vi "Write Recipe Data.vi"(8 "error in (no error)":errorcluster, 10 "Recipe Data":T1, 11 "Recipe Window in":refnum<class "Recipe Window.lvclass">) -> (0 "error out":errorcluster, 3 "Recipe Window out":refnum<class "Recipe Window.lvclass">)   [LabVIEW 2021, in "Recipe.lvlib" / "Recipe Window.lvclass"]
uses:
  Recipe Window.lvclass
  Typedefs/Recipe Data--cluster.ctl
  Recipe Window.lvclass/Recipe Window.ctl
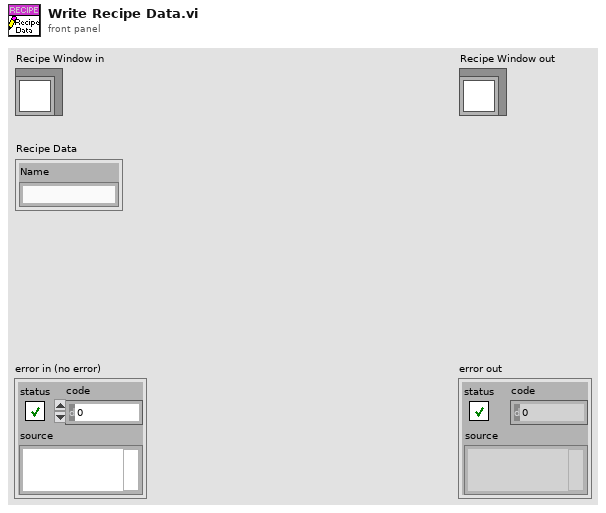
[diagram p1: front panel]
types:
  T1 = typedef "Recipe.lvlib/Recipe Window.lvclass/Recipe Data--cluster.ctl" = cluster{"Name":string}
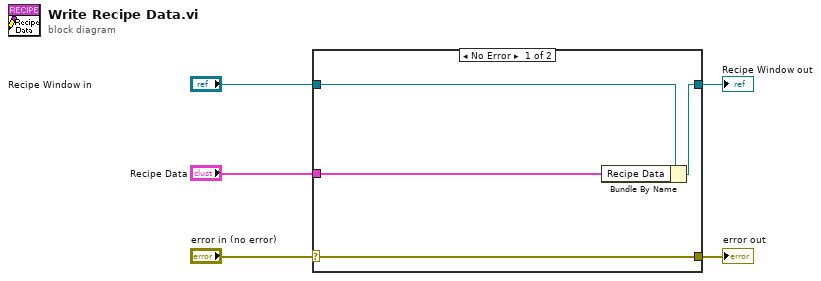
[diagram p0: block diagram]
diagram:
  n1 = case shown="No Error" "error in (no error)" {
    selector: "error in (no error)" -> [w9 w10]
    tunnel: [w9 w10] -> w4
    tunnel: [w7 w11] -> w2
    tunnel: "Recipe Window in" -> [w8 w11]
    tunnel: "Recipe Data" -> [w6 _]
    frame No Error {
      n2 = Bundle By Name(cluster=w8, "Recipe Data"=w6) -> (w7:refnum<class "Recipe Window.lvclass">)
    }
    frame Error {
    }
  }
  "error out" <- w4
  "Recipe Window out" <- w2
